vi "Get ListObj.vi"(8 "error in (no error)":errorcluster, 11 "StringList in":refnum<class "StringList.lvclass">) -> (0 "error out":errorcluster, 2 "List Object":refnum<class "ObjectList.lvclass">, 3 "StringList out":refnum<class "StringList.lvclass">)   [LabVIEW 2013, in "LapDog.Collections.v_.Lists.lvlib" / "StringList.lvclass"]
uses:
  StringList.lvclass
  ObjectList/ObjectList.lvclass
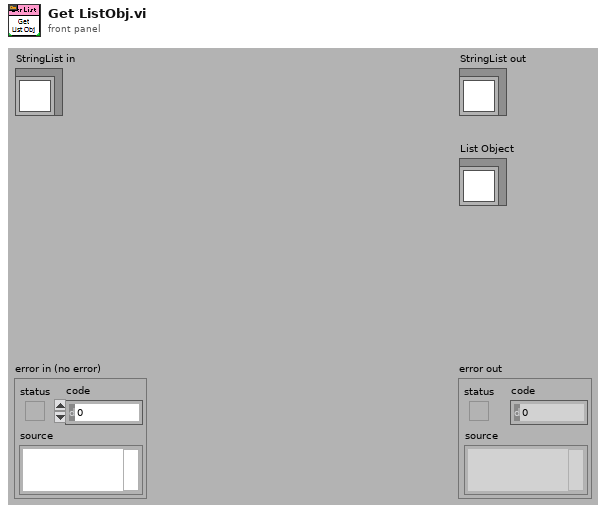
[diagram p1: front panel]
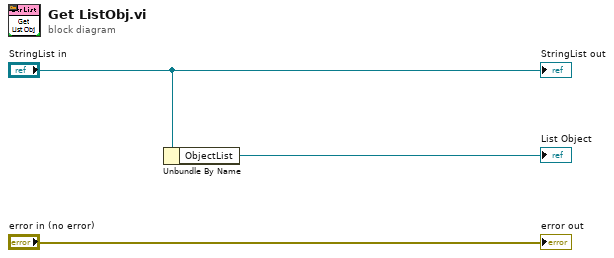
[diagram p0: block diagram]
diagram:
  n1 = Unbundle By Name("StringList in") -> ("ObjectList"=→"List Object":refnum<class "ObjectList.lvclass">)
  "error out" <- "error in (no error)"
  "StringList out" <- "StringList in"
